vi "FCO_Test.vi"() -> ()   [LabVIEW 2017]
uses:
  <vilib>/Instr/_visa.llb/VISA Configure Serial Port (Instr).vi
panel:
  in  "Delay Time (s)":dbl=0.15 caption="延迟时间(s)"
  in  "parity (0:none)":enum16{"None", "Odd", "Even", "Mark", "Space"}(ring)=enum."Even"
  in  "VISA resource name":refnum<visa-resource-name> caption="VISA资源名称"
  in  "port":u32
  out "读取缓冲区":string
  in  "停止":bool
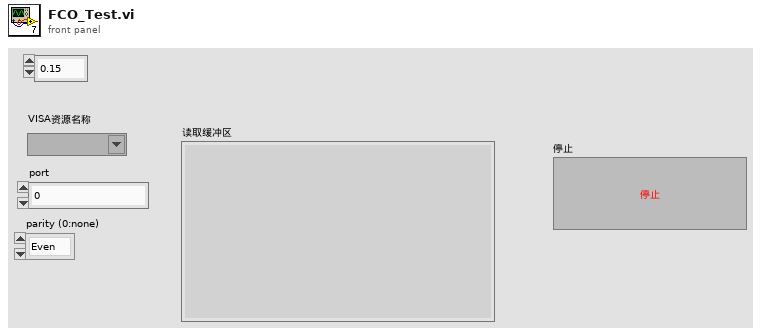
[diagram p1: front panel]
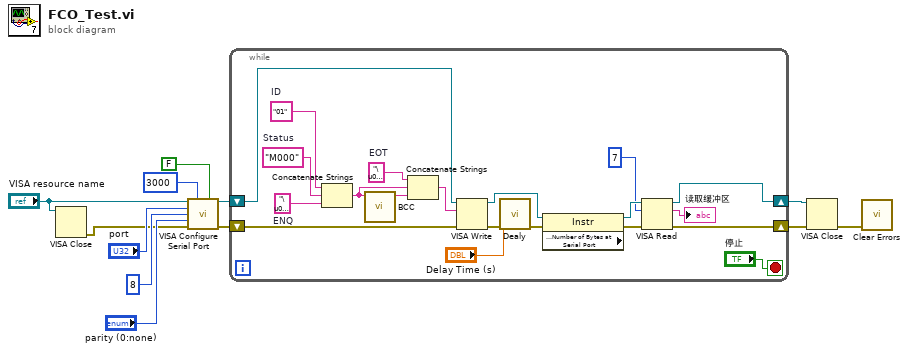
[diagram p0: block diagram]
diagram:
  n1 = VISA Close(VISA resource name="VISA resource name") -> (error out=w3:errorcluster)  [unwired: 1 in]
  n2 = call-poly "VISA Configure Serial Port"("VISA resource name"="VISA resource name", "timeout (10sec)"=u32 3000, "Enable Termination\nChar (T)"=FALSE ("Enable Termination\nChar (T)"), "baud rate (9600)"="port", "data bits (8)"=u16 8, "parity (0:none)"="parity (0:none)", "error in (no error)"=w3) -> ("VISA resource name out"=w8:refnum<visa-resource-name>, "error out"=w7:errorcluster)  [unwired: 2 in, 5 out]
  n3 = while {
    shift-right: [w19] -> w6
    shift-left: w8 -> [w20]
    shift-right: [w18] -> w5
    shift-left: w7 -> [w16]
    stop <- "停止" stop-if-true
    w13 = "01"  # ID
    w22 = "\u0005"  # ENQ
    w23 = "M000"  # Status
    w21 = "\u0004"  # EOT
    n4 = Concatenate Strings(w13, w23, w22) -> (w25:string)
    n5 = call "BCC.vi"("输入校验十六进制"=w25) -> ("BCC校验结果"=w24:string)  [unwired: 10 in]
    n6 = Concatenate Strings(w21, w25, w24) -> (w26:string)
    n7 = VISA Write(VISA resource name=w20, write buffer=w26, error in (no error)=w16) -> (VISA resource name out=w31:refnum<visa-resource-name>, error out=w30:errorcluster)  [unwired: 1 out]
    n8 = call "Dealy"("error in (no error)"=w30, "Delay Time (s)"="Delay Time (s)") -> ("error out"=w27:errorcluster)  [unwired: 9 in]
    n9 = property class="Instr" props=["Serial Settings:Number of Bytes at Serial Port"](reference=w31, error in=w27) -> (reference out=w29:refnum<visa-resource-name>, error out=w28:errorcluster)  [unwired: 1 out]
    n10 = VISA Read(VISA resource name=w29, byte count=u32 7 ("字节总数"), error in (no error)=w28) -> (VISA resource name out=w19:refnum<visa-resource-name>, read buffer=→"读取缓冲区":string, error out=w18:errorcluster)  [unwired: 1 out]
  }
  n11 = VISA Close(VISA resource name=w6, error in (no error)=w5) -> (error out=w2:errorcluster)
  n12 = call <vilib>:"Clear Errors.vi"("error in (no error)"=w2) -> ()  [unwired: 5 in, 2 out]
